vi "TW_BuildJSON.vi"(9 "Value":string, 10 "type":string, 11 "Thingworx":string) -> (2 "JSON":string, 3 "URL":string)   [LabVIEW 2019]
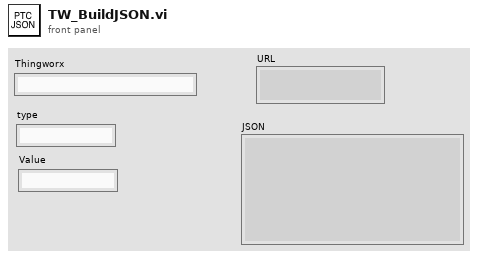
[diagram p1: front panel]
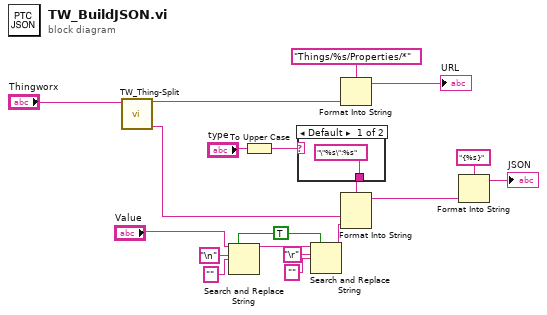
[diagram p0: block diagram]
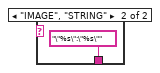
[diagram p2: hidden frame]
diagram:
  w16 = TRUE ("replace all? (F)")
  n1 = call "TW_Thing-Split.vi"("Property"="Thingworx") -> ("Property"=w1:string, "Thing"=w2:string)  [unwired: 9 in]
  n2 = Search and Replace String(replace all?=w16, input string="Value", search string="\n", replace string="" ("replace string (\"\")")) -> (result string=w14:string)  [unwired: 4 in, 3 out]
  n3 = To Upper Case(1:"type") -> (0:w9:string)
  n4 = case shown="Default" w9 {
    tunnel: ["\"%s\":%s" ("format string") "\"%s\":\"%s\"" ("format string")] -> w8
    frame Default {
    }
    frame "IMAGE", "STRING" {
    }
  }
  n5 = Search and Replace String(replace all?=w16, input string=w14, search string="\r", replace string="" ("replace string (\"\")")) -> (result string=w15:string)  [unwired: 4 in, 3 out]
  n6 = Format Into String(format string="Things/%s/Properties/*", w2) -> (resulting string=→"URL":string)  [unwired: 2 in, 1 out]
  n7 = Format Into String(format string=w8, w1, w15) -> (resulting string=w17:string)  [unwired: 2 in, 1 out]
  n8 = Format Into String(format string="{%s}", w17) -> (resulting string=→"JSON":string)  [unwired: 2 in, 1 out]
